vi "HumanDriveModeToNumb.vi"(11 "Human_DriveMode":T1) -> (3 "StateNumber":dbl)   [LabVIEW 2023]
uses:
  HumanDriveModeENUM.ctl
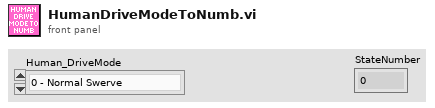
[diagram p1: front panel]
types:
  T1 = typedef "HumanDriveModeENUM.ctl" = enum16{"0 - Normal Swerve", "1 - Auto traj  - Left Speaker", "2 - Auto traj - Center Speaker", "3 - Auto traj - Speaker Right", "4 - Auto traj - Amp", "5 - Auto traj - Source", "6 - Auto traj -  Left Stage", "7 - Auto traj - Center Stage", "8 - Auto traj - Right Stage"}
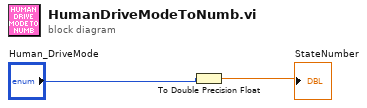
[diagram p0: block diagram]
diagram:
  n1 = To Double Precision Float(number="Human_DriveMode") -> (double precision float=→"StateNumber":dbl)
